vi "Untitled 14 (SubVI).vi"(9 "Кол-во выборок":i32, 10 "Filtered X":dbl[](array[numeric]), 11 "Пороговое значение in":dbl) -> (2 "Array":i16[](array[numeric]), 3 "Array 2":dbl[](array[numeric]))   [LabVIEW 2017]
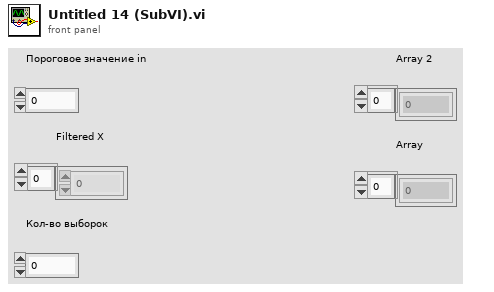
[diagram p1: front panel]
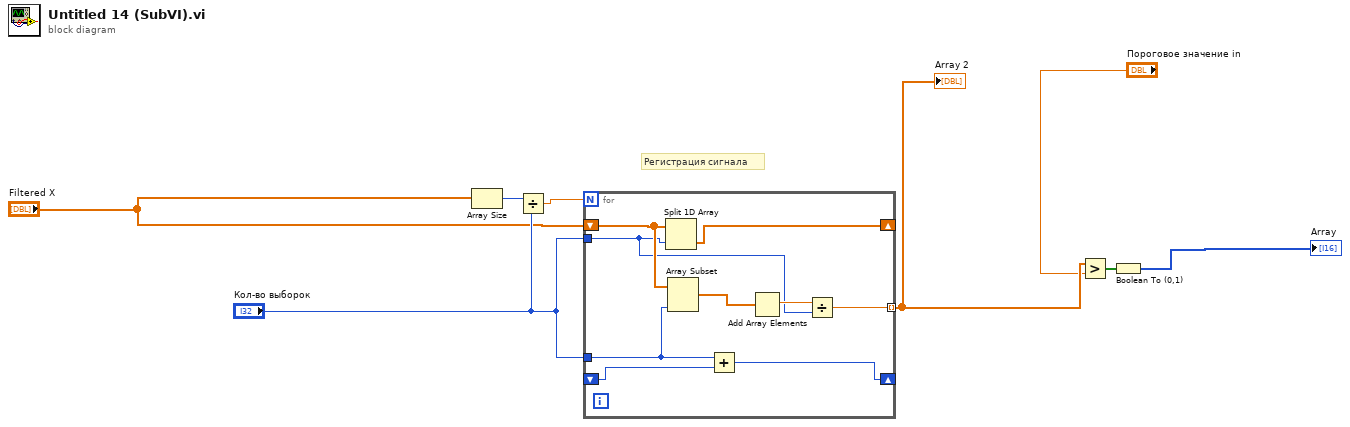
[diagram p0: block diagram]
diagram:
  # "Регистрация сигнала"
  n1 = Array Size(array="Filtered X") -> (size(s)=w1:i32)
  n2 = Divide(x=w1, y="Кол-во выборок") -> (x/y=w7:dbl)
  n3 = for {
    N: w7 -> [_]
    tunnel: "Кол-во выборок" -> [w10]
    shift-right: [w17] -> _
    shift-left: "Filtered X" -> [w16]
    tunnel: "Кол-во выборок" -> [w13]
    shift-right: [w14] -> _
    shift-left: _ -> [w15]
    tunnel: [w9] -> w5 mode=indexing
    n4 = Split 1D Array(array=w16, index=w10) -> (second subarray=w17:dbl[])  [unwired: 1 out]
    n5 = Array Subset(array=w16, length=w13) -> (w12:dbl[])  [unwired: 1 in]
    n6 = Add(x=w13, y=w15) -> (x+y=w14:i32)
    n7 = Add Array Elements(numeric array=w12) -> (sum=w11:dbl)
    n8 = Divide(x=w11, y=w10) -> (x/y=w9:dbl)
  }
  "Array 2" <- w5
  n9 = Greater?(x=w5, y="Пороговое значение in") -> (0:w6:bool[])
  n10 = Boolean To (0,1)(Boolean=w6) -> (0, 1=→"Array":i16[])
